vi "Server.vi"() -> ()   [LabVIEW 2020]
panel:
  in  "file path (use dialog)":path
  out "zone6":bool
  out "zone5":bool
  out "zone4":bool
  out "zone3":bool
  out "zone2":bool
  out "zone1":bool
  # "Green = Normal\nRed = Alarm\nBlue = Bypass\nOrange = Tamper"
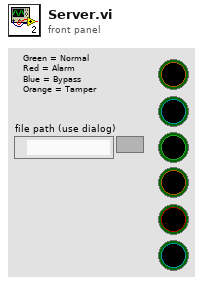
[diagram p1: front panel]
types:
  T1 = enum16{"open", "replace", "create", "open or create", "replace or create", "replace or create with confirmation"}
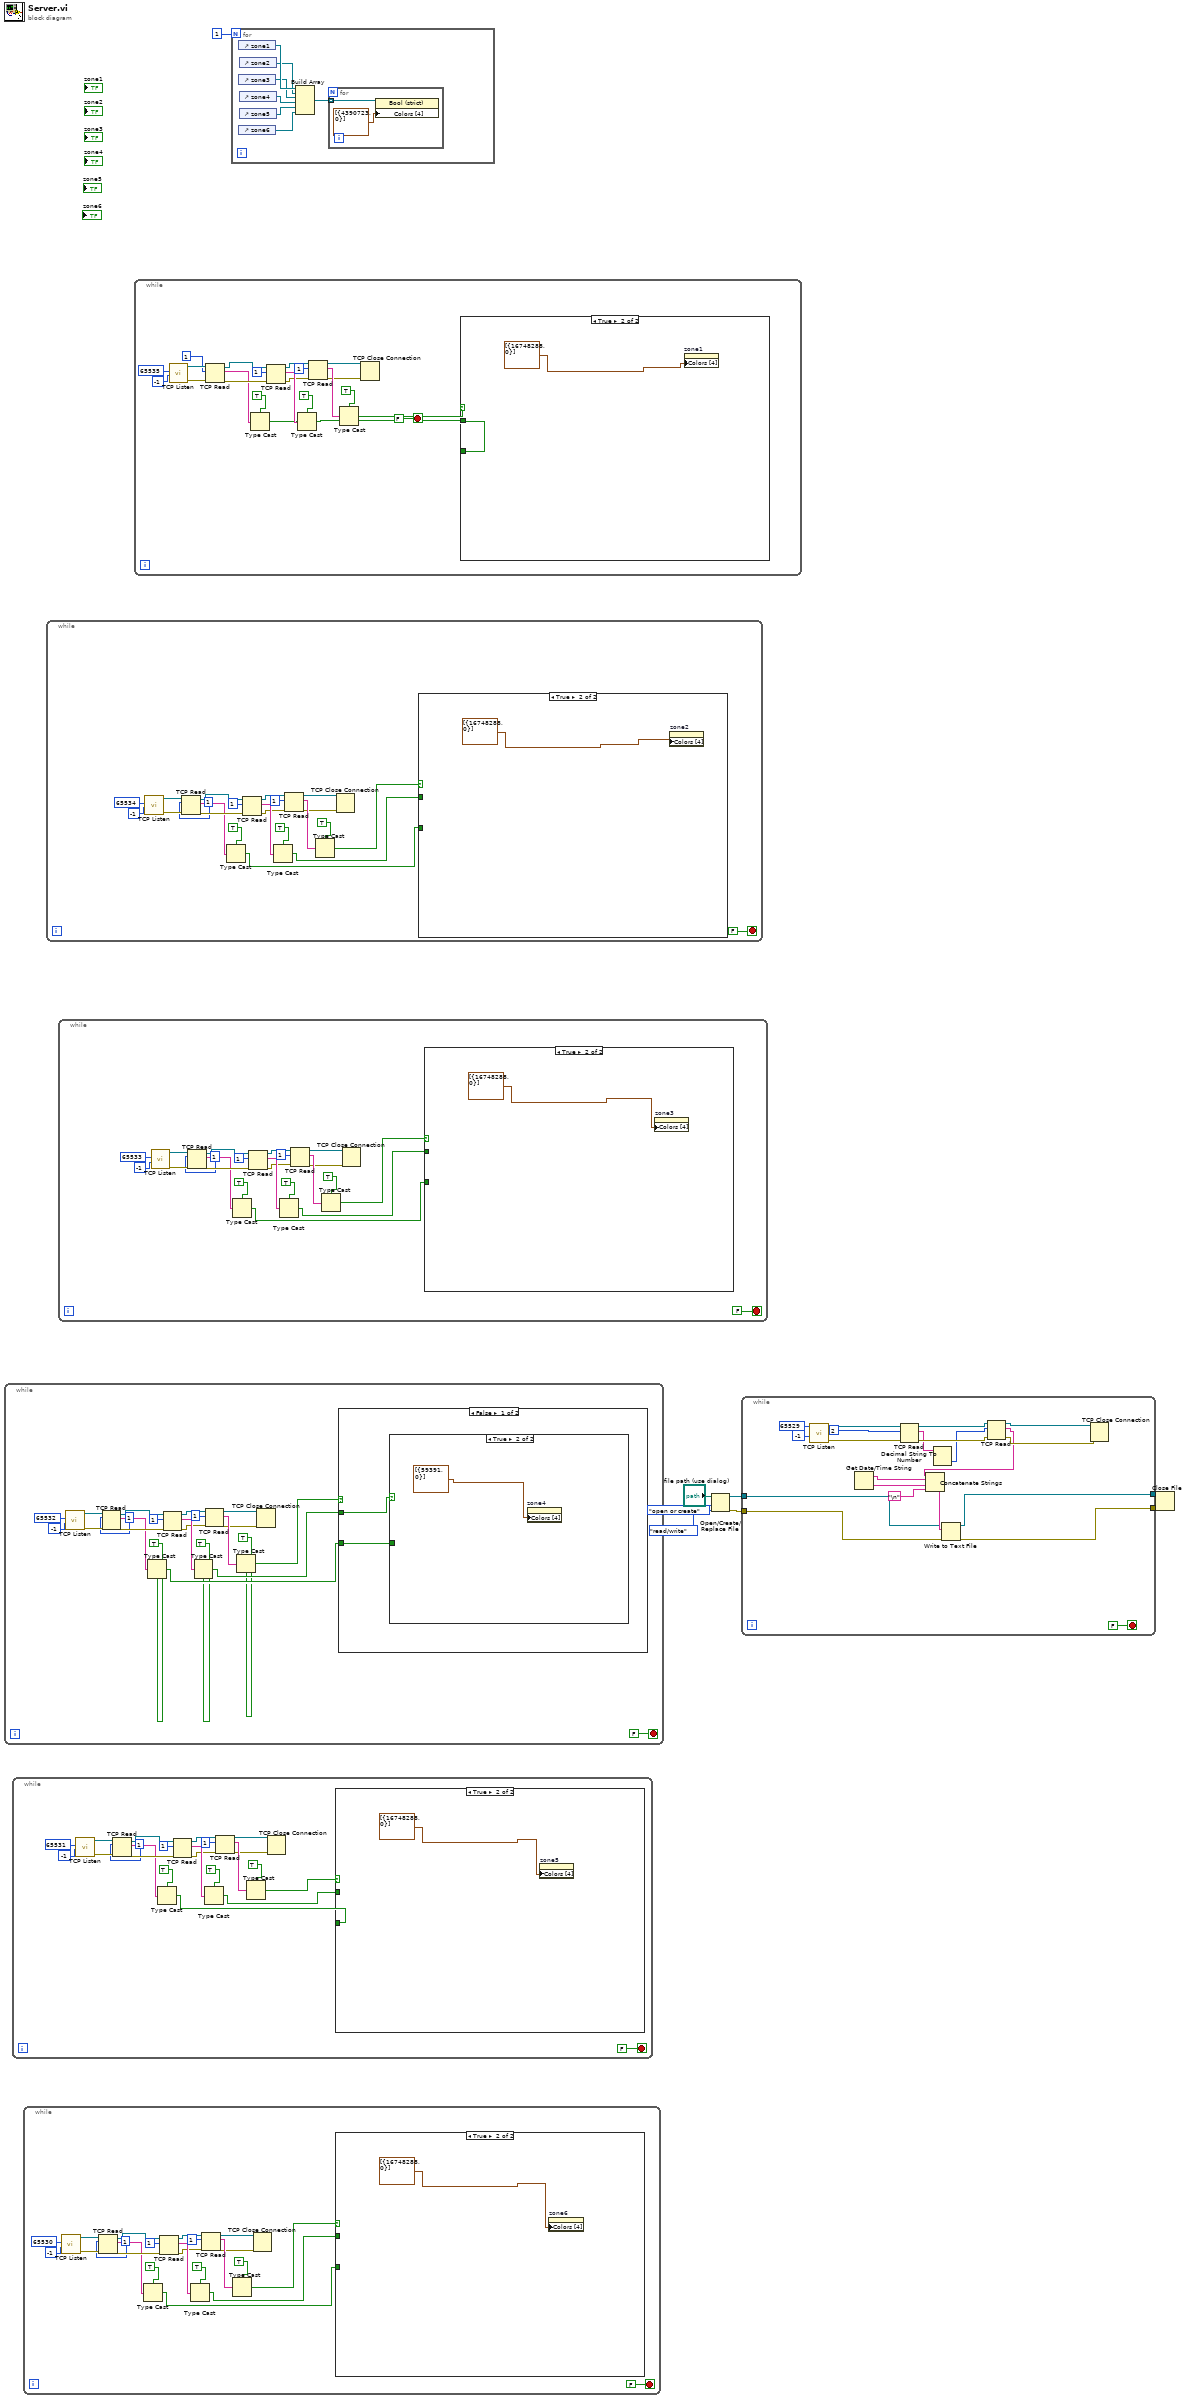
[diagram p0: block diagram]
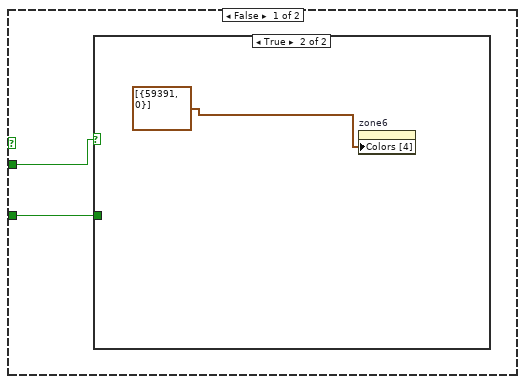
[diagram p2: hidden frame]
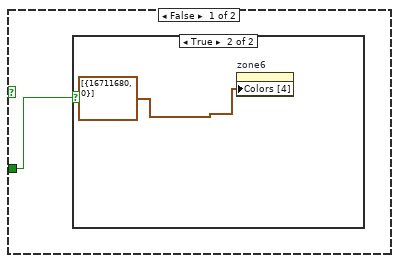
[diagram p3: hidden frame]
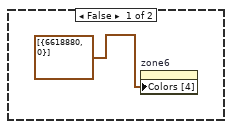
[diagram p4: hidden frame]
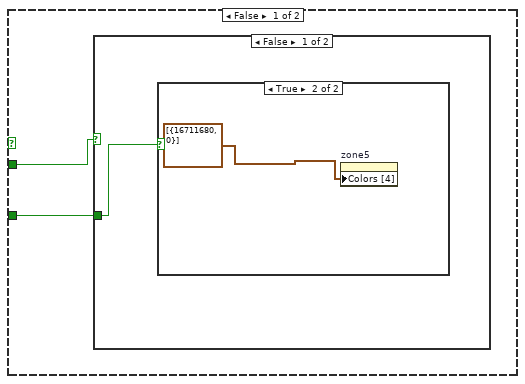
[diagram p5: hidden frame]
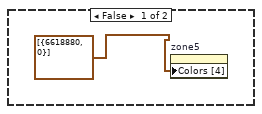
[diagram p6: hidden frame]
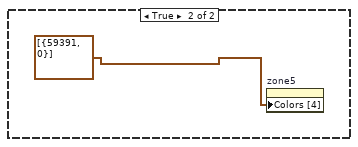
[diagram p7: hidden frame]
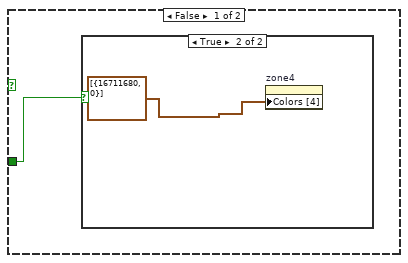
[diagram p8: hidden frame]
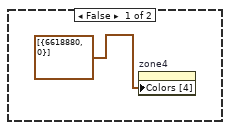
[diagram p9: hidden frame]
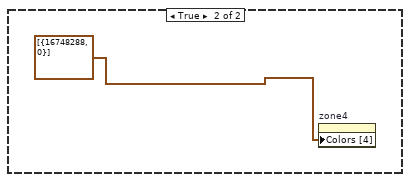
[diagram p10: hidden frame]
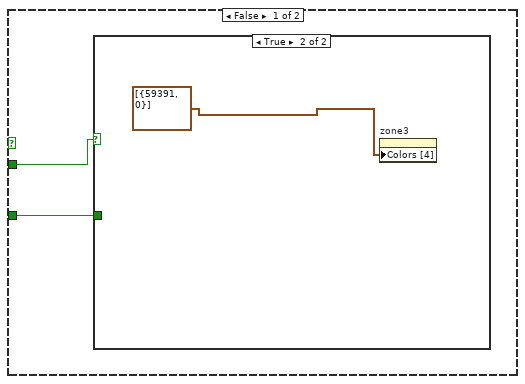
[diagram p11: hidden frame]
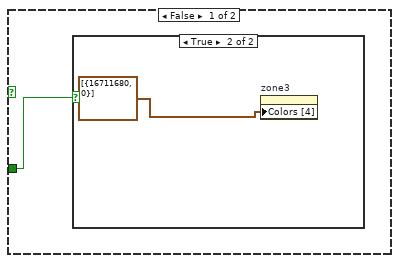
[diagram p12: hidden frame]
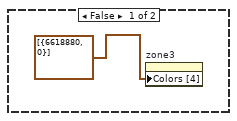
[diagram p13: hidden frame]
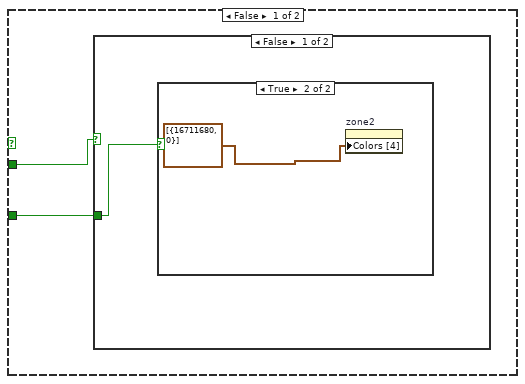
[diagram p14: hidden frame]
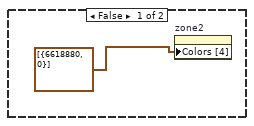
[diagram p15: hidden frame]
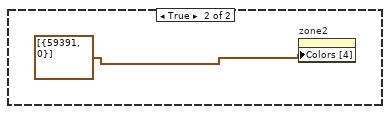
[diagram p16: hidden frame]
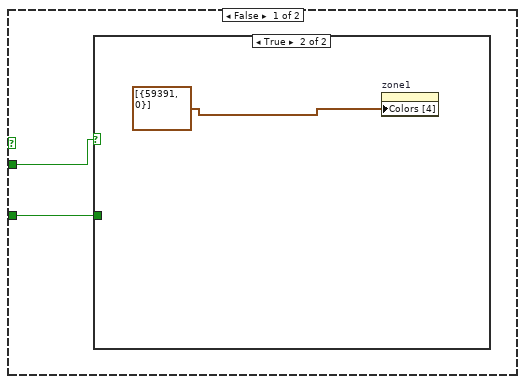
[diagram p17: hidden frame]
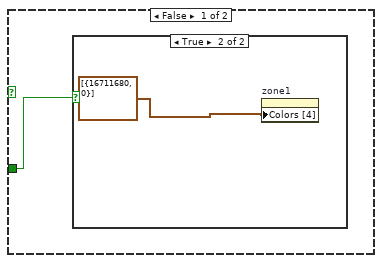
[diagram p18: hidden frame]
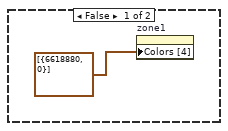
[diagram p19: hidden frame]
diagram:
  n1 = while {
    stop <- FALSE stop-if-true
    n2 = call <vilib>:"TCP Listen.vi"("timeout ms (wait forever: -1)"=-1, "port"=u16 65532) -> ("error out"=w20:errorcluster, "connection ID"=w19:refnum<k5>)  [unwired: 5 in, 3 out]
    n3 = TCP Read(connection ID=w19, bytes to read=1, error in (no error)=w20) -> (connection ID out=w21:refnum<k5>, data out=w18:string, error out=w22:errorcluster)  [unwired: 2 in]
    n4 = Type Cast(type=TRUE, x=w18) -> (*(type *) &x=w31:bool)
    n5 = TCP Read(connection ID=w21, bytes to read=1, error in (no error)=w22) -> (connection ID out=w24:refnum<k5>, data out=w28:string, error out=w23:errorcluster)  [unwired: 2 in]
    n6 = Type Cast(type=TRUE, x=w28) -> (*(type *) &x=w30:bool)
    n7 = TCP Read(connection ID=w24, bytes to read=1, error in (no error)=w23) -> (connection ID out=w25:refnum<k5>, data out=w27:string, error out=w26:errorcluster)  [unwired: 2 in]
    n8 = Type Cast(type=TRUE, x=w27) -> (*(type *) &x=w29:bool)
    n9 = TCP Close Connection(connection ID=w25, error in (no error)=w26) -> ()  [unwired: 1 in, 2 out]
    n10 = case shown="False" w29 {
      tunnel: w30 -> [w33 _]
      tunnel: w31 -> [w32 _]
      frame False {
        n11 = case shown="True" w33 {
          tunnel: w32 -> [w34 _]
          frame False {
            n12 = case shown="True" w34 {
              frame False {
                n13 = property on="zone4" class="Bool (strict)"("Colors [4]"=cluster{u32, i32}[] [{6618880, 0}]) -> ()  [unwired: 2 in, 2 out]
              }
              frame True {
                n14 = property on="zone4" class="Bool (strict)"("Colors [4]"=cluster{u32, i32}[] [{16711680, 0}]) -> ()  [unwired: 2 in, 2 out]
              }
            }
          }
          frame True {
            n15 = property on="zone4" class="Bool (strict)"("Colors [4]"=cluster{u32, i32}[] [{59391, 0}]) -> ()  [unwired: 2 in, 2 out]
          }
        }
      }
      frame True {
        n16 = property on="zone4" class="Bool (strict)"("Colors [4]"=cluster{u32, i32}[] [{16748288, 0}]) -> ()  [unwired: 2 in, 2 out]
      }
    }
  }
  n17 = while {
    stop <- FALSE stop-if-true
    n18 = call <vilib>:"TCP Listen.vi"("timeout ms (wait forever: -1)"=-1, "port"=u16 65531) -> ("error out"=w50:errorcluster, "connection ID"=w49:refnum<k5>)  [unwired: 5 in, 3 out]
    n19 = TCP Read(connection ID=w49, bytes to read=1, error in (no error)=w50) -> (connection ID out=w51:refnum<k5>, data out=w48:string, error out=w52:errorcluster)  [unwired: 2 in]
    n20 = Type Cast(type=TRUE, x=w48) -> (*(type *) &x=w61:bool)
    n21 = TCP Read(connection ID=w51, bytes to read=1, error in (no error)=w52) -> (connection ID out=w54:refnum<k5>, data out=w58:string, error out=w53:errorcluster)  [unwired: 2 in]
    n22 = Type Cast(type=TRUE, x=w58) -> (*(type *) &x=w60:bool)
    n23 = TCP Read(connection ID=w54, bytes to read=1, error in (no error)=w53) -> (connection ID out=w55:refnum<k5>, data out=w57:string, error out=w56:errorcluster)  [unwired: 2 in]
    n24 = Type Cast(type=TRUE, x=w57) -> (*(type *) &x=w59:bool)
    n25 = TCP Close Connection(connection ID=w55, error in (no error)=w56) -> ()  [unwired: 1 in, 2 out]
    n26 = case shown="True" w59 {
      tunnel: w60 -> [w63 _]
      tunnel: w61 -> [w62 _]
      frame False {
        n27 = case shown="False" w63 {
          tunnel: w62 -> [w64 _]
          frame False {
            n28 = case shown="True" w64 {
              frame False {
                n29 = property on="zone5" class="Bool (strict)"("Colors [4]"=cluster{u32, i32}[] [{6618880, 0}]) -> ()  [unwired: 2 in, 2 out]
              }
              frame True {
                n30 = property on="zone5" class="Bool (strict)"("Colors [4]"=cluster{u32, i32}[] [{16711680, 0}]) -> ()  [unwired: 2 in, 2 out]
              }
            }
          }
          frame True {
            n31 = property on="zone5" class="Bool (strict)"("Colors [4]"=cluster{u32, i32}[] [{59391, 0}]) -> ()  [unwired: 2 in, 2 out]
          }
        }
      }
      frame True {
        n32 = property on="zone5" class="Bool (strict)"("Colors [4]"=cluster{u32, i32}[] [{16748288, 0}]) -> ()  [unwired: 2 in, 2 out]
      }
    }
  }
  n33 = while {
    stop <- FALSE stop-if-true
    n34 = call <vilib>:"TCP Listen.vi"("timeout ms (wait forever: -1)"=-1, "port"=u16 65530) -> ("error out"=w80:errorcluster, "connection ID"=w79:refnum<k5>)  [unwired: 5 in, 3 out]
    n35 = TCP Read(connection ID=w79, bytes to read=1, error in (no error)=w80) -> (connection ID out=w81:refnum<k5>, data out=w78:string, error out=w82:errorcluster)  [unwired: 2 in]
    n36 = Type Cast(type=TRUE, x=w78) -> (*(type *) &x=w91:bool)
    n37 = TCP Read(connection ID=w81, bytes to read=1, error in (no error)=w82) -> (connection ID out=w84:refnum<k5>, data out=w88:string, error out=w83:errorcluster)  [unwired: 2 in]
    n38 = Type Cast(type=TRUE, x=w88) -> (*(type *) &x=w90:bool)
    n39 = TCP Read(connection ID=w84, bytes to read=1, error in (no error)=w83) -> (connection ID out=w85:refnum<k5>, data out=w87:string, error out=w86:errorcluster)  [unwired: 2 in]
    n40 = Type Cast(type=TRUE, x=w87) -> (*(type *) &x=w89:bool)
    n41 = TCP Close Connection(connection ID=w85, error in (no error)=w86) -> ()  [unwired: 1 in, 2 out]
    n42 = case shown="True" w89 {
      tunnel: w90 -> [w93 _]
      tunnel: w91 -> [w92 _]
      frame False {
        n43 = case shown="True" w93 {
          tunnel: w92 -> [w94 _]
          frame False {
            n44 = case shown="True" w94 {
              frame False {
                n45 = property on="zone6" class="Bool (strict)"("Colors [4]"=cluster{u32, i32}[] [{6618880, 0}]) -> ()  [unwired: 2 in, 2 out]
              }
              frame True {
                n46 = property on="zone6" class="Bool (strict)"("Colors [4]"=cluster{u32, i32}[] [{16711680, 0}]) -> ()  [unwired: 2 in, 2 out]
              }
            }
          }
          frame True {
            n47 = property on="zone6" class="Bool (strict)"("Colors [4]"=cluster{u32, i32}[] [{59391, 0}]) -> ()  [unwired: 2 in, 2 out]
          }
        }
      }
      frame True {
        n48 = property on="zone6" class="Bool (strict)"("Colors [4]"=cluster{u32, i32}[] [{16748288, 0}]) -> ()  [unwired: 2 in, 2 out]
      }
    }
  }
  n49 = while {
    stop <- FALSE stop-if-true
    n50 = call <vilib>:"TCP Listen.vi"("timeout ms (wait forever: -1)"=-1, "port"=u16 65534) -> ("error out"=w110:errorcluster, "connection ID"=w109:refnum<k5>)  [unwired: 5 in, 3 out]
    n51 = TCP Read(connection ID=w109, bytes to read=1, error in (no error)=w110) -> (connection ID out=w111:refnum<k5>, data out=w108:string, error out=w112:errorcluster)  [unwired: 2 in]
    n52 = Type Cast(type=TRUE, x=w108) -> (*(type *) &x=w121:bool)
    n53 = TCP Read(connection ID=w111, bytes to read=1, error in (no error)=w112) -> (connection ID out=w114:refnum<k5>, data out=w118:string, error out=w113:errorcluster)  [unwired: 2 in]
    n54 = Type Cast(type=TRUE, x=w118) -> (*(type *) &x=w120:bool)
    n55 = TCP Read(connection ID=w114, bytes to read=1, error in (no error)=w113) -> (connection ID out=w115:refnum<k5>, data out=w117:string, error out=w116:errorcluster)  [unwired: 2 in]
    n56 = Type Cast(type=TRUE, x=w117) -> (*(type *) &x=w119:bool)
    n57 = TCP Close Connection(connection ID=w115, error in (no error)=w116) -> ()  [unwired: 1 in, 2 out]
    n58 = case shown="True" w119 {
      tunnel: w120 -> [w123 _]
      tunnel: w121 -> [w122 _]
      frame False {
        n59 = case shown="False" w123 {
          tunnel: w122 -> [w124 _]
          frame False {
            n60 = case shown="True" w124 {
              frame False {
                n61 = property on="zone2" class="Bool (strict)"("Colors [4]"=cluster{u32, i32}[] [{6618880, 0}]) -> ()  [unwired: 2 in, 2 out]
              }
              frame True {
                n62 = property on="zone2" class="Bool (strict)"("Colors [4]"=cluster{u32, i32}[] [{16711680, 0}]) -> ()  [unwired: 2 in, 2 out]
              }
            }
          }
          frame True {
            n63 = property on="zone2" class="Bool (strict)"("Colors [4]"=cluster{u32, i32}[] [{59391, 0}]) -> ()  [unwired: 2 in, 2 out]
          }
        }
      }
      frame True {
        n64 = property on="zone2" class="Bool (strict)"("Colors [4]"=cluster{u32, i32}[] [{16748288, 0}]) -> ()  [unwired: 2 in, 2 out]
      }
    }
  }
  n65 = while {
    stop <- FALSE stop-if-true
    n66 = call <vilib>:"TCP Listen.vi"("timeout ms (wait forever: -1)"=-1, "port"=u16 65533) -> ("error out"=w140:errorcluster, "connection ID"=w139:refnum<k5>)  [unwired: 5 in, 3 out]
    n67 = TCP Read(connection ID=w139, bytes to read=1, error in (no error)=w140) -> (connection ID out=w141:refnum<k5>, data out=w138:string, error out=w142:errorcluster)  [unwired: 2 in]
    n68 = Type Cast(type=TRUE, x=w138) -> (*(type *) &x=w151:bool)
    n69 = TCP Read(connection ID=w141, bytes to read=1, error in (no error)=w142) -> (connection ID out=w144:refnum<k5>, data out=w148:string, error out=w143:errorcluster)  [unwired: 2 in]
    n70 = Type Cast(type=TRUE, x=w148) -> (*(type *) &x=w150:bool)
    n71 = TCP Read(connection ID=w144, bytes to read=1, error in (no error)=w143) -> (connection ID out=w145:refnum<k5>, data out=w147:string, error out=w146:errorcluster)  [unwired: 2 in]
    n72 = Type Cast(type=TRUE, x=w147) -> (*(type *) &x=w149:bool)
    n73 = TCP Close Connection(connection ID=w145, error in (no error)=w146) -> ()  [unwired: 1 in, 2 out]
    n74 = case shown="True" w149 {
      tunnel: w150 -> [w153 _]
      tunnel: w151 -> [w152 _]
      frame False {
        n75 = case shown="True" w153 {
          tunnel: w152 -> [w154 _]
          frame False {
            n76 = case shown="True" w154 {
              frame False {
                n77 = property on="zone3" class="Bool (strict)"("Colors [4]"=cluster{u32, i32}[] [{6618880, 0}]) -> ()  [unwired: 2 in, 2 out]
              }
              frame True {
                n78 = property on="zone3" class="Bool (strict)"("Colors [4]"=cluster{u32, i32}[] [{16711680, 0}]) -> ()  [unwired: 2 in, 2 out]
              }
            }
          }
          frame True {
            n79 = property on="zone3" class="Bool (strict)"("Colors [4]"=cluster{u32, i32}[] [{59391, 0}]) -> ()  [unwired: 2 in, 2 out]
          }
        }
      }
      frame True {
        n80 = property on="zone3" class="Bool (strict)"("Colors [4]"=cluster{u32, i32}[] [{16748288, 0}]) -> ()  [unwired: 2 in, 2 out]
      }
    }
  }
  n81 = while {
    stop <- FALSE stop-if-true
    n82 = call <vilib>:"TCP Listen.vi"("timeout ms (wait forever: -1)"=-1, "port"=u16 65535) -> ("error out"=w169:errorcluster, "connection ID"=w168:refnum<k5>)  [unwired: 5 in, 3 out]
    n83 = TCP Read(connection ID=w168, bytes to read=1, error in (no error)=w169) -> (connection ID out=w171:refnum<k5>, data out=w167:string, error out=w172:errorcluster)  [unwired: 2 in]
    n84 = Type Cast(type=TRUE, x=w167) -> (*(type *) &x=w170:bool)
    n85 = TCP Read(connection ID=w171, bytes to read=1, error in (no error)=w172) -> (connection ID out=w174:refnum<k5>, data out=w177:string, error out=w173:errorcluster)  [unwired: 2 in]
    n86 = Type Cast(type=TRUE, x=w177) -> (*(type *) &x=w178:bool)
    n87 = TCP Read(connection ID=w174, bytes to read=1, error in (no error)=w173) -> (connection ID out=w175:refnum<k5>, data out=w179:string, error out=w176:errorcluster)  [unwired: 2 in]
    n88 = Type Cast(type=TRUE, x=w179) -> (*(type *) &x=w180:bool)
    n89 = TCP Close Connection(connection ID=w175, error in (no error)=w176) -> ()  [unwired: 1 in, 2 out]
    n90 = case shown="True" w180 {
      tunnel: w178 -> [w183 _]
      tunnel: w170 -> [w182 _]
      frame False {
        n91 = case shown="True" w183 {
          tunnel: w182 -> [w184 _]
          frame False {
            n92 = case shown="True" w184 {
              frame False {
                n93 = property on="zone1" class="Bool (strict)"("Colors [4]"=cluster{u32, i32}[] [{6618880, 0}]) -> ()  [unwired: 2 in, 2 out]
              }
              frame True {
                n94 = property on="zone1" class="Bool (strict)"("Colors [4]"=cluster{u32, i32}[] [{16711680, 0}]) -> ()  [unwired: 2 in, 2 out]
              }
            }
          }
          frame True {
            n95 = property on="zone1" class="Bool (strict)"("Colors [4]"=cluster{u32, i32}[] [{59391, 0}]) -> ()  [unwired: 2 in, 2 out]
          }
        }
      }
      frame True {
        n96 = property on="zone1" class="Bool (strict)"("Colors [4]"=cluster{u32, i32}[] [{16748288, 0}]) -> ()  [unwired: 2 in, 2 out]
      }
    }
  }
  n97 = for {
    N: 1 -> [_]
    n98 = control-ref of="zone1"() -> (w194:refnum<vi>)
    n99 = control-ref of="zone3"() -> (w192:refnum<vi>)
    n100 = control-ref of="zone6"() -> (w189:refnum<vi>)
    n101 = control-ref of="zone2"() -> (w193:refnum<vi>)
    n102 = control-ref of="zone4"() -> (w191:refnum<vi>)
    n103 = control-ref of="zone5"() -> (w190:refnum<vi>)
    n104 = Build Array "Build Array"(w194, w193, w192, w191, w190, w189) -> (w195:refnum<vi>[])
    n105 = for {
      tunnel: w195 -> [w196] mode=indexing
      n106 = property class="Bool (strict)"(reference=w196, "Colors [4]"=cluster{u32, u32}[] [{4390723, 0}] ("Couleurs [4]")) -> ()  [unwired: 1 in, 2 out]
    }
  }
  n107 = Open/Create/Replace File(file path (use dialog)="file path (use dialog)", operation (0:open)=T1."open or create", access (0:read/write)=enum16{"read/write", "read-only", "write-only"}."read/write") -> (refnum out=w6:refnum<file>, error out=w7:errorcluster)  [unwired: 3 in, 1 out]
  n108 = while {
    tunnel: w7 -> [w205]
    tunnel: w6 -> [w206]
    tunnel: [w207] -> w5
    tunnel: [w208] -> w4
    stop <- FALSE stop-if-true
    n109 = call <vilib>:"TCP Listen.vi"("timeout ms (wait forever: -1)"=-1, "port"=u16 65529) -> ("error out"=w217:errorcluster, "connection ID"=w216:refnum<k5>)  [unwired: 5 in, 3 out]
    n110 = Get Date/Time String() -> (date string=w210:string, time string=w213:string)  [unwired: 3 in]
    n111 = TCP Read(connection ID=w216, bytes to read=2, error in (no error)=w217) -> (connection ID out=w204:refnum<k5>, data out=w200:string, error out=w203:errorcluster)  [unwired: 2 in]
    n112 = Decimal String To Number(string=w200) -> (number=w199:i32)  [unwired: 2 in, 1 out]
    n113 = TCP Read(connection ID=w204, bytes to read=w199, error in (no error)=w203) -> (connection ID out=w201:refnum<k5>, data out=w198:string, error out=w202:errorcluster)  [unwired: 2 in]
    n114 = Concatenate Strings(w198, w210, w213, "\n") -> (w211:string)
    n115 = Write to Text File(file (use dialog)=w206, text=w211, error in=w205) -> (refnum out=w208:refnum<file>, error out=w207:errorcluster)  [unwired: 1 in, 1 out]
    n116 = TCP Close Connection(connection ID=w201, error in (no error)=w202) -> ()  [unwired: 1 in, 2 out]
  }
  n117 = Close File(refnum=w4, error in=w5) -> ()  [unwired: 2 out]
